vi "Send Observe Data Msg.vi"(8 "error in (no error)":errorcluster, 9 "Publication Time (Use Current Time)":timestamp, 10 "Value":variant, 11 "Observe Data Msg":refnum<class "Observe Data Msg.lvclass">) -> (0 "error out":errorcluster)   [LabVIEW 2018, in "MVA Framework.lvlib" / "IObserver.lvlib" / "Observe Data Msg.lvclass"]
doc: "发送观察数据消息"
uses:
  Observe Data Msg.lvclass
  composed-af-messages/Source/RoundTripMessage/RoundTripMessage.lvclass
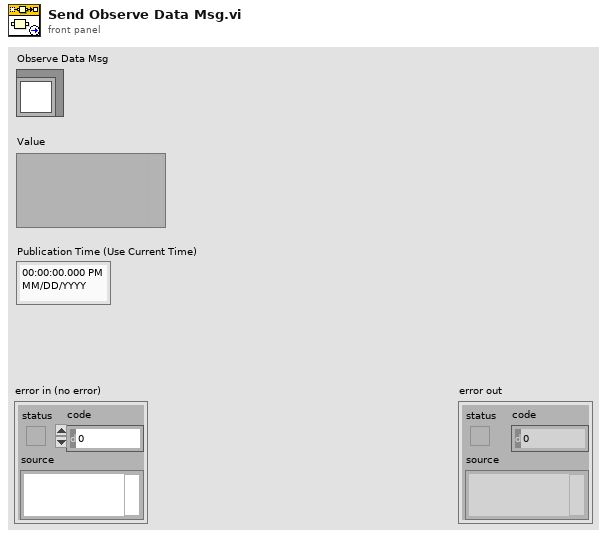
[diagram p1: front panel]
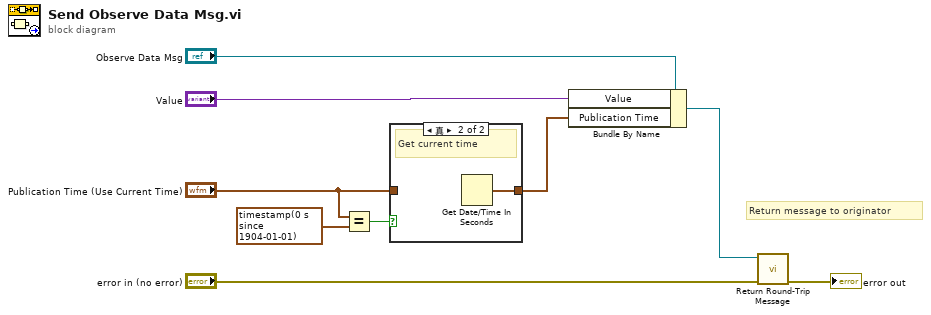
[diagram p0: block diagram]
diagram:
  # "Return message to originator"
  n1 = Equal?(x="Publication Time (Use Current Time)", y=timestamp(0 s since 1904-01-01)) -> (x = y?=w4:bool)
  n2 = case shown="真" w4 {
    tunnel: "Publication Time (Use Current Time)" -> [w10 _]
    tunnel: [w10 w11] -> w2
    frame False {
      # "Use input time"
    }
    frame True {
      # "Get current time"
      n3 = Get Date/Time In Seconds() -> (seconds since 1Jan1904=w11:timestamp)
    }
  }
  n4 = Bundle By Name(cluster="Observe Data Msg", "Value"="Value", "Publication Time"=w2) -> (w6:refnum<class "Observe Data Msg.lvclass">)
  n5 = call "Return Round-Trip Message.vi"("error in (no error)"="error in (no error)", "RoundTripMessage In"=w6) -> ("error out"=→"error out":errorcluster)  [unwired: 9 in]
